vi "EL-RIO-CM v1.0 Open Throughput AI (N Samples).vi"(7 "Allow multiple opens?":bool, 8 "error in (no error)":errorcluster, 10 "Channel Names":string[](array[string]), 11 "Resource name":T7 caption="RIO Device") -> (0 "error out":errorcluster, 1 "AI (N Samples) Scale Constants List":T1, 2 "AI (N Samples) Channel List":T3, 3 "myRIO Ref Out":T5 caption="EL-RIO-CM Ref Out")   [LabVIEW 2021]
uses:
  <vilib>/userDefined/High Color/nirio_resource_hc.ctl
  <vilib>/myRIO/Common/Instrument Driver Framework/Utilities/typedefs/myRIO v1.0 Reference.ctl
  <vilib>/myRIO/Common/Instrument Driver Framework/Utilities/typedefs/Generic FPGA Reference.ctl
  <vilib>/myRIO/Common/Instrument Driver Framework/myRIO v1.0/AI Block/typedefs/AI Block Channels List.ctl
  <vilib>/myRIO/Common/Instrument Driver Framework/myRIO v1.0/AI Block/typedefs/AI Block Channels Enum.ctl
  <vilib>/myRIO/Common/Instrument Driver Framework/Utilities/typedefs/Analog Scaling Constants List.ctl
  <vilib>/myRIO/Common/Instrument Driver Framework/Utilities/typedefs/Analog Scaling Constants.ctl
  <vilib>/myRIO/Common/Instrument Driver Framework/EL-RIO-CM v1.0/AI Block/typedefs/EL-RIO-CM v1.0 AI Block Channels Enum.ctl
  <vilib>/Utility/VariantDataType/GetNumericInfo.vi
  <vilib>/Utility/error.llb/Error Cluster From Error Code.vi
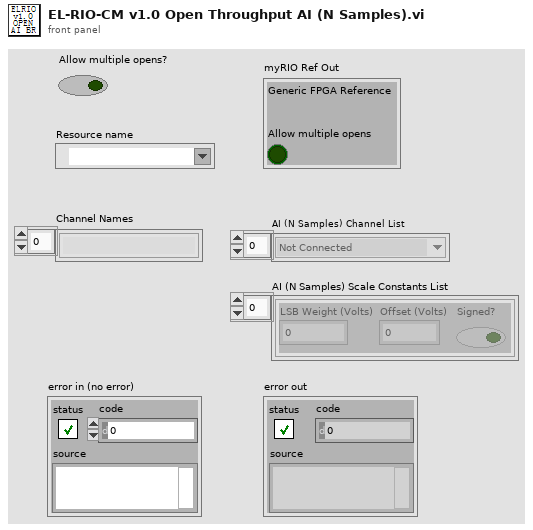
[diagram p1: front panel]
types:
  T1 = typedef "Analog Scaling Constants List.ctl" = T2[]
  T2 = typedef "Analog Scaling Constants.ctl" = cluster{"LSB Weight (Volts)":dbl, "Offset (Volts)":dbl, "Signed?":bool}
  T3 = typedef "AI Block Channels List.ctl" = T4[]
  T4 = typedef "AI Block Channels Enum.ctl" = enum16{"Not Connected", "A/AI0 (N Samples)", "A/AI1 (N Samples)", "A/AI2 (N Samples)", "A/AI3 (N Samples)", "A/AI4 (N Samples)", "A/AI5 (N Samples)", "A/AI6 (N Samples)", "A/AI7 (N Samples)", "A/AI0 (DIFF N Samples)", "A/AI1 (DIFF N Samples)", "A/AI2 (DIFF N Samples)", "A/AI3 (DIFF N Samples)", "B/AI0 (N Samples)", "B/AI1 (N Samples)", "B/AI2 (N Samples)", "B/AI3 (N Samples)", "B/AI4 (N Samples)", "B/AI5 (N Samples)", "B/AI6 (N Samples)", "B/AI7 (N Samples)", "B/AI0 (DIFF N Samples)", "B/AI1 (DIFF N Samples)", "B/AI2 (DIFF N Samples)", "B/AI3 (DIFF N Samples)"}
  T5 = typedef "myRIO v1.0 Reference.ctl" = cluster{"Generic FPGA Reference":T6, "Allow multiple opens":bool}
  T6 = typedef "Generic FPGA Reference.ctl" = refnum<k20>
  T7 = typedef "nirio_resource_hc.ctl" = tag
  T8 = typedef "EL-RIO-CM v1.0 AI Block Channels Enum.ctl" = enum16{"Not Connected", "A/AI0 (N Samples)"}
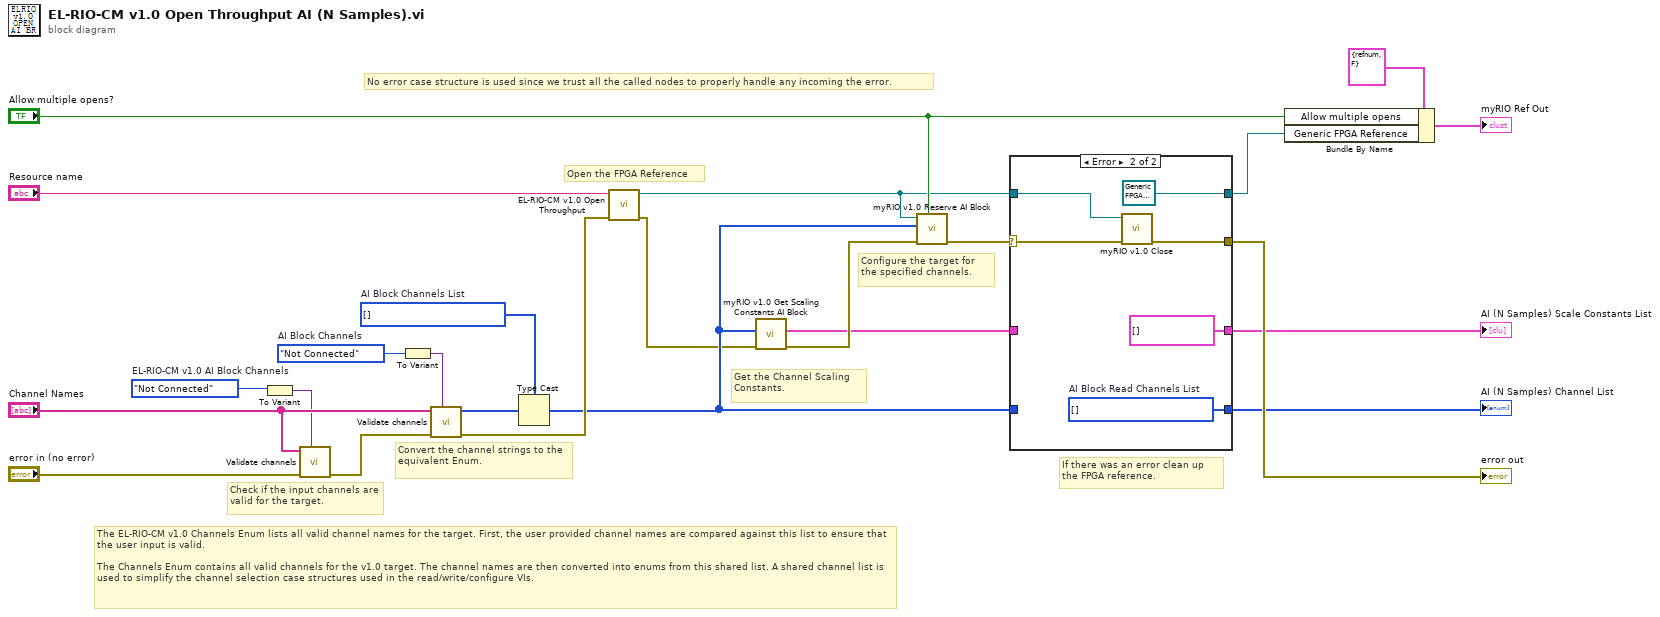
[diagram p0: block diagram]
diagram:
  w1 = EL-RIO-CM_v1.0_AI_Block_Channels_Enum."Not Connected"  # EL-RIO-CM v1.0 AI Block Channels
  w11 = T3 [] items=["Not Connected", "A/AI0 (N Samples)", "A/AI1 (N Samples)", "A/AI2 (N Samples)", "A/AI3 (N Samples)", "A/AI4 (N Samples)", "A/AI5 (N Samples)", "A/AI6 (N Samples)", "A/AI7 (N Samples)", "A/AI0 (DIFF N Samples)", "A/AI1 (DIFF N Samples)", "A/AI2 (DIFF N Samples)", "A/AI3 (DIFF N Samples)", "B/AI0 (N Samples)", "B/AI1 (N Samples)", "B/AI2 (N Samples)", "B/AI3 (N Samples)", "B/AI4 (N Samples)", "B/AI5 (N Samples)", "B/AI6 (N Samples)", "B/AI7 (N Samples)", "B/AI0 (DIFF N Samples)", "B/AI1 (DIFF N Samples)", "B/AI2 (DIFF N Samples)", "B/AI3 (DIFF N Samples)"]  # AI Block Channels List
  w12 = AI_Block_Channels_Enum."Not Connected"  # AI Block Channels
  # "Get the Channel Scaling Constants."
  # "The EL-RIO-CM v1.0 Channels Enum lists all valid channel names for the target. First, the user provided channel names are compared against this list to ensure that the user input is valid.\n\nThe Channels Enum contains all valid channels for the v1.0 target. The channel names are then converted into enums from this shared list. A shared channel list is used to simplify the channel selection case structures used in the read/write/configure VIs."
  # "If there was an error clean up the FPGA reference."
  # "Configure the target for the specified channels."
  # "Open the FPGA Reference"
  # "No error case structure is used since we trust all the called nodes to properly handle any incoming the error."
  # "Convert the channel strings to the equivalent Enum."
  # "Check if the input channels are valid for the target."
  n1 = To Variant(anything=w1) -> (Variant=w13:variant)
  n2 = call <vilib>:"Validate channels.vi"("Channels Enum Variant"=w13, "error in (no error)"="error in (no error)", "Channel Names"="Channel Names") -> ("error out"=w23:errorcluster)  [unwired: 7 in, 1 out]
  n3 = To Variant(anything=w12) -> (Variant=w14:variant)
  n4 = call <vilib>:"Validate channels.vi"("Channels Enum Variant"=w14, "error in (no error)"=w23, "Channel Names"="Channel Names") -> ("error out"=w19:errorcluster, "Index Array"=w18:u16[])  [unwired: 7 in]
  n5 = Type Cast(type=w11, x=w18) -> (*(type *) &x=w7:T3)
  n6 = call <vilib>:"EL-RIO-CM v1.0 Open Throughput.vi"("error in (no error)"=w19, "Resource name"="Resource name") -> ("error out"=w6:errorcluster, "myRIO FPGA Ref Out"=w2:T6)  [unwired: 8 in]
  n7 = call <vilib>:"myRIO v1.0 Get Scaling Constants AI Block.vi"("error in (no error)"=w6, "AI (N Samples) Channels List"=w7) -> ("error out"=w5:errorcluster, "Scale Constants Array"=w4:T1)  [unwired: 8 in]
  n8 = call <vilib>:"myRIO v1.0 Reserve AI Block.vi"("Allow multiple opens?"="Allow multiple opens?", "error in (no error)"=w5, "AI (N Samples) Channels List"=w7, "Generic FPGA Reference"=w2) -> ("error out"=w15:errorcluster)  [unwired: 7 in]
  n9 = case shown="Error" w15 {
    selector: w15 -> [w28 w34]
    tunnel: [w26 T6 refnum ("EL-RIO-CM FPGA Ref Out")] -> w17
    tunnel: [w28 w33] -> w21
    tunnel: [w27 w30] -> w10
    tunnel: w7 -> [w27 _]
    tunnel: w2 -> [w26 w31]
    tunnel: w4 -> [w25 _]
    tunnel: [w25 T1 [] ("Scale Constants Array")] -> w3
    frame No Error {
    }
    frame Error {
      w30 = T3 [] items=["Not Connected", "A/AI0 (N Samples)", "A/AI1 (N Samples)", "A/AI2 (N Samples)", "A/AI3 (N Samples)", "A/AI4 (N Samples)", "A/AI5 (N Samples)", "A/AI6 (N Samples)", "A/AI7 (N Samples)", "A/AI0 (DIFF N Samples)", "A/AI1 (DIFF N Samples)", "A/AI2 (DIFF N Samples)", "A/AI3 (DIFF N Samples)", "B/AI0 (N Samples)", "B/AI1 (N Samples)", "B/AI2 (N Samples)", "B/AI3 (N Samples)", "B/AI4 (N Samples)", "B/AI5 (N Samples)", "B/AI6 (N Samples)", "B/AI7 (N Samples)", "B/AI0 (DIFF N Samples)", "B/AI1 (DIFF N Samples)", "B/AI2 (DIFF N Samples)", "B/AI3 (DIFF N Samples)"]  # AI Block Read Channels List
      n10 = call <vilib>:"myRIO v1.0 Close.vi"("error in (no error)"=w34, "myRIO FPGA Ref In"=w31) -> ("error out"=w33:errorcluster)  [unwired: 9 in]
    }
  }
  "error out" <- w21
  "AI (N Samples) Channel List" <- w10
  "AI (N Samples) Scale Constants List" <- w3
  n11 = Bundle By Name(cluster=T5 {"Generic FPGA Reference"=refnum, "Allow multiple opens"=FALSE} ("EL-RIO-CM Ref Out"), "Allow multiple opens"="Allow multiple opens?", "Generic FPGA Reference"=w17) -> (→"myRIO Ref Out":T5)
